vi "OPA.SetShutterState.vi"(8 "error in (no error)":errorcluster, 10 "Shutter State":bool, 11 "OPA.OrpheusHP in":refnum<class "OPA.OrpheusHP.lvclass">) -> (0 "error out":errorcluster, 3 "OPA.OrpheusHP out":refnum<class "OPA.OrpheusHP.lvclass">)   [LabVIEW 2019, in "OPA.OrpheusHP.lvclass"]
uses:
  OPA.OrpheusHP.lvclass
  E:/UPWORK/Laser Tool/Topas4PublicAPI/NET_SDK/Topas4Lib.dll
  Topas4PublicAPI/NET_SDK/Topas4Lib.dll
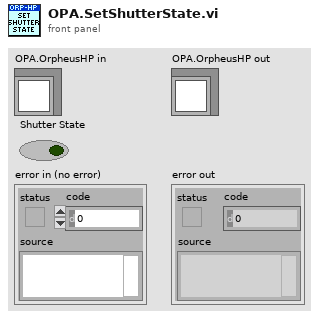
[diagram p1: front panel]
types:
  T1 = typedef "OPA.OrpheusHP.lvclass/Resource--Cluster.ctl" = cluster{"TopasDevice":refnum<k24>, "WavelengthService":refnum<k24>, "ShutterService":refnum<k24>}
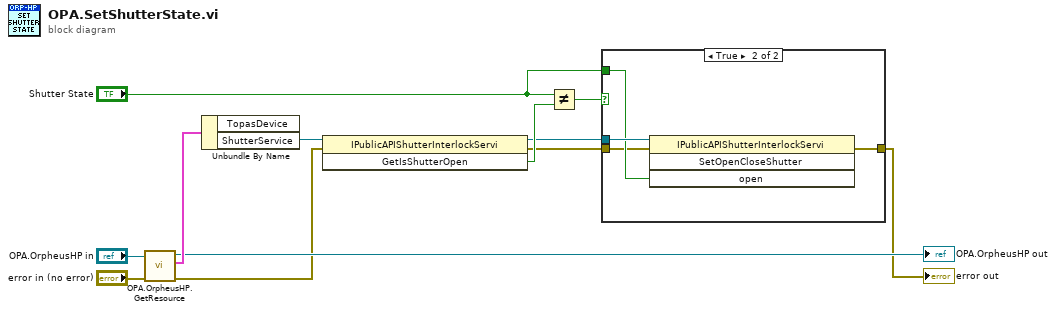
[diagram p0: block diagram]
diagram:
  n1 = call "OPA.OrpheusHP.GetResource.vi"("error in (no error)"="error in (no error)", "OPA.OrpheusHP in"="OPA.OrpheusHP in") -> ("error out"=w3:errorcluster, "Resource"=w10:T1, "OPA.OrpheusHP out"=→"OPA.OrpheusHP out":refnum<class "OPA.OrpheusHP.lvclass">)  [unwired: 7 in]
  n2 = Unbundle By Name(w10) -> ("ShutterService"=w9:refnum<k24>)  [unwired: 1 out]
  n3 = invoke class="IPublicAPIShutterInterlockServi" method="GetIsShutterOpen"(reference=w9, error in=w3) -> (reference out=w6:refnum<k24>, error out=w2:errorcluster, "GetIsShutterOpen"=w8:bool)  [unwired: 1 in]
  n4 = Not Equal?(x="Shutter State", y=w8) -> (x != y?=w7:bool)
  n5 = case shown="True" w7 {
    tunnel: w6 -> [_ w17]
    tunnel: "Shutter State" -> [_ w16]
    tunnel: w2 -> [w13 w15]
    tunnel: [w13 w14] -> w1
    frame False {
    }
    frame True {
      n6 = invoke class="IPublicAPIShutterInterlockServi" method="SetOpenCloseShutter"(reference=w17, error in=w15, "open"=w16) -> (error out=w14:errorcluster)  [unwired: 1 in, 3 out]
    }
  }
  "error out" <- w1
